vi "application_compress.vi"(6 "distribution_folder":path, 8 "error in (no error)":errorcluster, 11 "build_specifications":T1) -> (0 "error out":errorcluster)   [LabVIEW 2015, in "lv-builder-default.lvlib"]
uses:
  lv-builder-default.lvlib
  lv-build/public/_controls/build_specification.ctl
  lv-build/public/_controls/build_type.ctl
  <userlib>/antonio-alexander/lv-bin-7zip/public/api/v1/advanced/compress_exe.vi
  <userlib>/antonio-alexander/lv-bin-7zip/public/api/v1/v1.lvlib
  lv-build/lv-build.lvlib
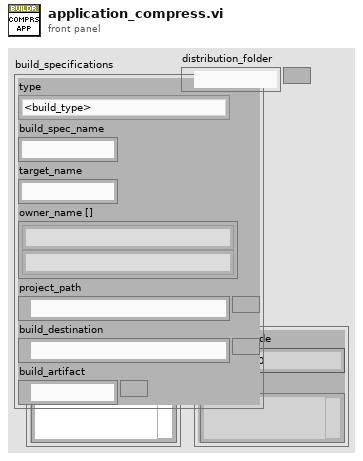
[diagram p1: front panel]
types:
  T1 = typedef "lv-build.lvlib/build_specification.ctl" = cluster{"type":T2, "build_spec_name":string, "target_name":string, "owner_name []":string[], "project_path":path, "build_destination":path, "build_artifact":path}
  T2 = typedef "lv-build.lvlib/build_type.ctl" = enum16{"<build_type>", "application_pc", "application_rt", "installer", "llb", "lvlibp", "zip", "fpga", "<null>"}
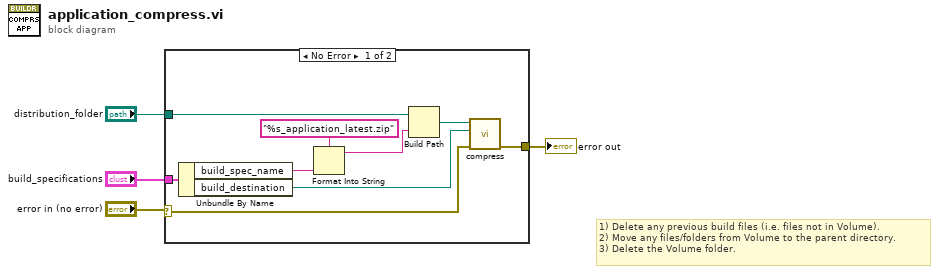
[diagram p0: block diagram]
diagram:
  # "1) Delete any previous build files (i.e. files not in Volume).\n2) Move any files/folders from Volume to the parent directory. \n3) Delete the Volume folder."
  n1 = case shown="No Error" "error in (no error)" {
    selector: "error in (no error)" -> [w6 w14]
    tunnel: "build_specifications" -> [w13 _]
    tunnel: [w7 w14] -> w2
    tunnel: "distribution_folder" -> [w5 _]
    frame No Error {
      n2 = Unbundle By Name(w13) -> ("build_spec_name"=w11:string, "build_destination"=w9:path)
      n3 = Format Into String(format string="%s_application_latest.zip", w11) -> (resulting string=w10:string)  [unwired: 2 in, 1 out]
      n4 = Build Path(base path=w5, name or relative path=w10) -> (appended path=w8:path)
      n5 = call-poly <userlib>:"compress.vi"("error in (no error)"=w6, "files_to_add"=w9, "archive_path in"=w8) -> ("error out"=w7:errorcluster)  [unwired: 7 in, 1 out]
    }
    frame Error {
    }
  }
  "error out" <- w2
